vi "channel front panel validation.vi"() -> (0 "invalid_channel_class test":bool, 1 "invalid_channel_type test":bool, 2 "missing_channel_test":bool, 3 "valid channel test":bool)   [LabVIEW 2014, in "UI reference module tests.lvlib"]
uses:
  UI reference module tests.lvlib
  <vilib>/NI/Tag Bus/tag/Data Type.ctl
  <vilib>/NI/Tag Bus Module Framework/channel/channel classification.ctl
  <vilib>/NI/Tag Bus Module Framework/channel/TBM channel.lvclass
  module/execution/UI Reference runtime old.lvclass
  <vilib>/NI/Tag Bus/tag/tag descriptor.lvclass
panel:
  in  "invalid_channel_class":dbl
  in  "valid_channel_name_2":dbl
  in  "invalid_channel_type":string
  in  "valid_channel_name":dbl
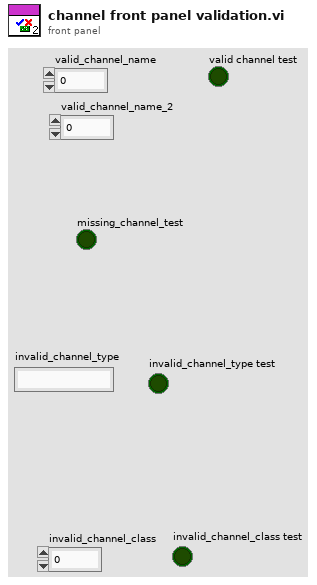
[diagram p1: front panel]
types:
  T1 = typedef "tag bus.lvlib/tag descriptor.lvclass/Data Type.ctl" = enum16{"Double", "Single", "I64", "I32", "I16", "I8", "U64", "U32", "U16", "U8", "Boolean", "String", "Array of Double", "Array of Single", "Array of I64", "Array of I32", "Array of I16", "Array of I8", "Array of U64", "Array of U32", "Array of U16", "Array of U8", "Array of Boolean", "Array of String"}
  T2 = typedef "TBM channel.lvclass/channel classification.ctl" = enum16{"input data", "output data", "processing parameter", "processing result"}
  T3 = cluster{"channel name":string, "data type":T1, "channel classification":T2}[]
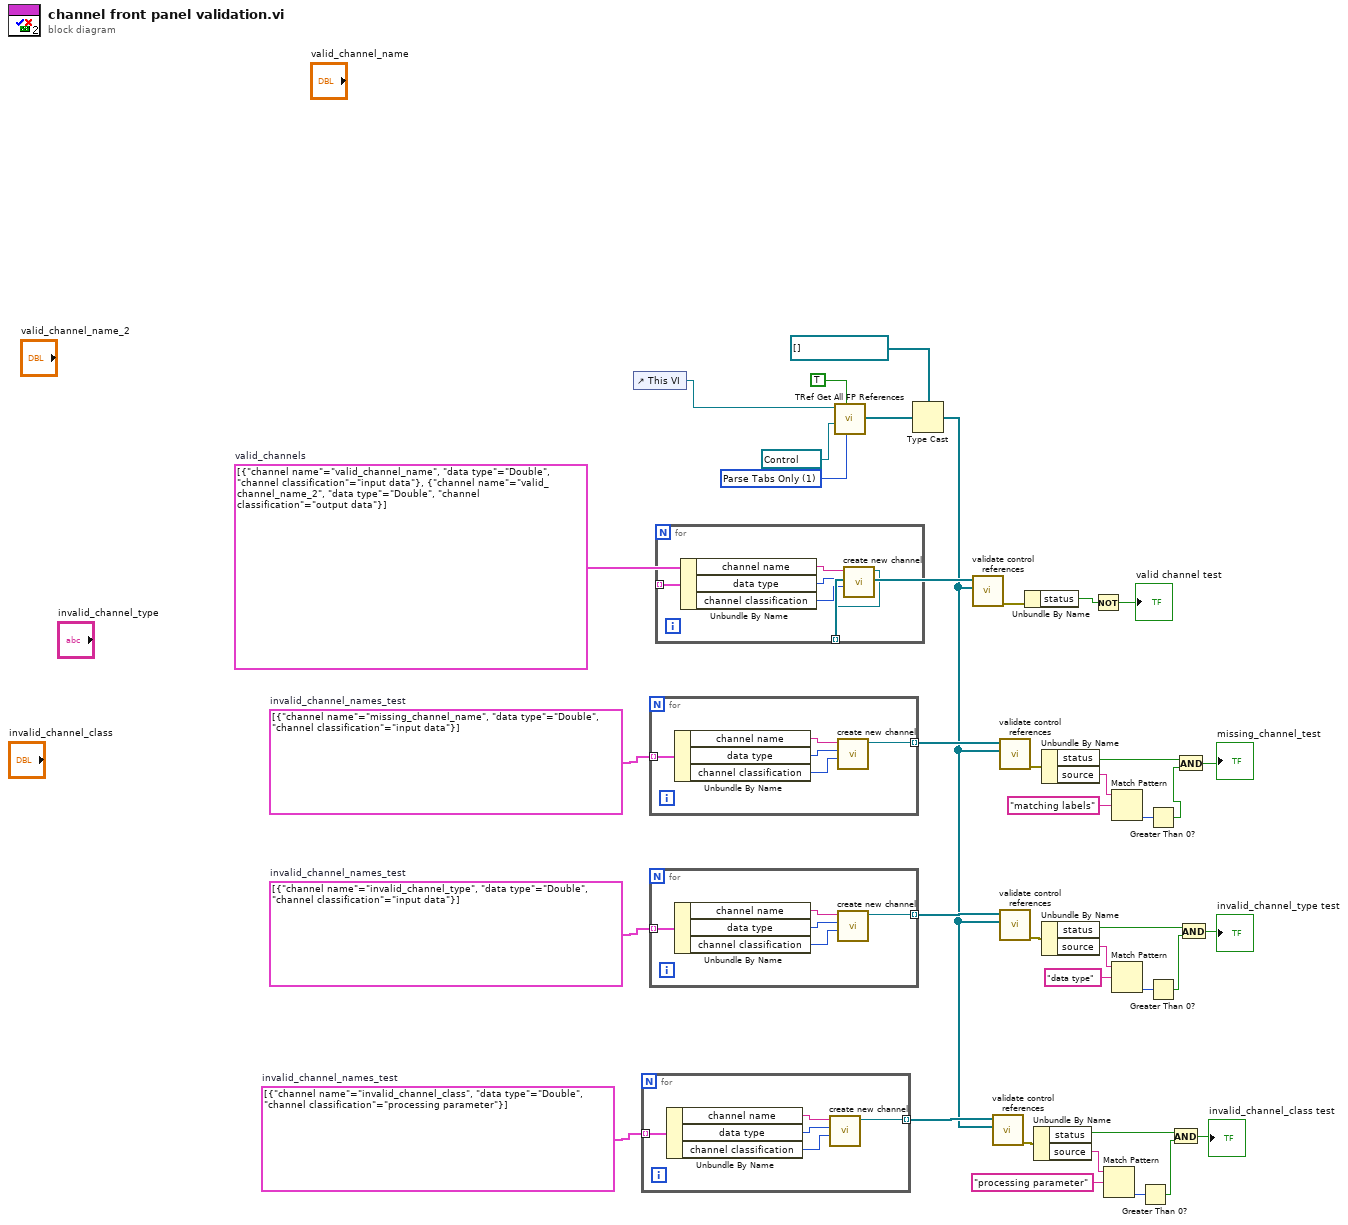
[diagram p0: block diagram]
diagram:
  w7 = T3 [{"channel name"="invalid_channel_class", "data type"=enum."Double", "channel classification"=enum."processing parameter"}]  # invalid_channel_names_test
  w17 = T3 [{"channel name"="invalid_channel_type", "data type"=enum."Double", "channel classification"=enum."input data"}]  # invalid_channel_names_test
  w28 = T3 [{"channel name"="missing_channel_name", "data type"=enum."Double", "channel classification"=enum."input data"}]  # invalid_channel_names_test
  w33 = T3 [{"channel name"="valid_channel_name", "data type"=enum."Double", "channel classification"=enum."input data"}, {"channel name"="valid_channel_name_2", "data type"=enum."Double", "channel classification"=enum."output data"}]  # valid_channels
  w38 = u16 1 items=["Parse All", "Parse Tabs Only"] ("Parsing Rule")
  n1 = control-ref of="This VI"() -> (w34:refnum<vi>)
  n2 = for {
    tunnel: w7 -> [w41] mode=indexing
    tunnel: [w40] -> w5 mode=indexing
    n3 = Unbundle By Name(w41) -> ("channel name"=w44:string, "data type"=w43:T1, "channel classification"=w42:T2)
    n4 = call <vilib>:"create new channel.vi"("channel classification"=w42, "data type"=w43, "channel name"=w44) -> ("channel"=w40:refnum<class "TBM channel.lvclass">)  [unwired: 8 in]
  }
  n5 = for {
    tunnel: w28 -> [w46] mode=indexing
    tunnel: [w45] -> w26 mode=indexing
    n6 = Unbundle By Name(w46) -> ("channel name"=w49:string, "data type"=w48:T1, "channel classification"=w47:T2)
    n7 = call <vilib>:"create new channel.vi"("channel classification"=w47, "data type"=w48, "channel name"=w49) -> ("channel"=w45:refnum<class "TBM channel.lvclass">)  [unwired: 8 in]
  }
  n8 = for {
    tunnel: w17 -> [w51] mode=indexing
    tunnel: [w50] -> w19 mode=indexing
    n9 = Unbundle By Name(w51) -> ("channel name"=w54:string, "data type"=w53:T1, "channel classification"=w52:T2)
    n10 = call <vilib>:"create new channel.vi"("channel classification"=w52, "data type"=w53, "channel name"=w54) -> ("channel"=w50:refnum<class "TBM channel.lvclass">)  [unwired: 8 in]
  }
  n11 = for {
    tunnel: w33 -> [w56] mode=indexing
    tunnel: [w55] -> w32 mode=indexing
    n12 = Unbundle By Name(w56) -> ("channel name"=w59:string, "data type"=w58:T1, "channel classification"=w57:T2)
    n13 = call <vilib>:"create new channel.vi"("channel classification"=w57, "data type"=w58, "channel name"=w59) -> ("channel"=w55:refnum<class "TBM channel.lvclass">)  [unwired: 8 in]
  }
  n14 = call <vilib>:"TRef Get All FP References.vi"("Parsing Rule"=w38, "Ignore Decorations?"=TRUE, "GObj Refnum"=refnum<vi> refnum ("Ctl Refnum"), "VI Refnum"=w34) -> ("All FP Objects"=w36:refnum<vi>[])  [unwired: 3 in, 4 out]
  n15 = Type Cast(type=refnum<vi>[] [] ("front panel elements in"), x=w36) -> (*(type *) &x=w1:refnum<vi>[])
  n16 = call "validate control references.vi"("front panel elements in"=w1, "channels in"=w32) -> ("error out"=w31:errorcluster)  [unwired: 9 in]
  n17 = call "validate control references.vi"("front panel elements in"=w1, "channels in"=w5) -> ("error out"=w6:errorcluster)  [unwired: 9 in]
  n18 = call "validate control references.vi"("front panel elements in"=w1, "channels in"=w26) -> ("error out"=w27:errorcluster)  [unwired: 9 in]
  n19 = call "validate control references.vi"("front panel elements in"=w1, "channels in"=w19) -> ("error out"=w18:errorcluster)  [unwired: 9 in]
  n20 = Unbundle By Name(w31) -> ("status"=w30:bool)
  n21 = Unbundle By Name(w6) -> ("status"=w9:bool, "source"=w4:string)
  n22 = Unbundle By Name(w27) -> ("status"=w16:bool, "source"=w25:string)
  n23 = Unbundle By Name(w18) -> ("status"=w12:bool, "source"=w20:string)
  n24 = Not(x=w30) -> (.not. x?=→"valid channel test":bool)
  n25 = Match Pattern(string=w4, regular expression="processing parameter") -> (offset past match=w2:i32)  [unwired: 1 in, 3 out]
  n26 = Match Pattern(string=w25, regular expression="matching labels") -> (offset past match=w23:i32)  [unwired: 1 in, 3 out]
  n27 = Match Pattern(string=w20, regular expression="data type") -> (offset past match=w22:i32)  [unwired: 1 in, 3 out]
  n28 = Greater Than 0?(x=w2) -> (x > 0?=w10:bool)
  n29 = Greater Than 0?(x=w23) -> (x > 0?=w15:bool)
  n30 = Greater Than 0?(x=w22) -> (x > 0?=w11:bool)
  n31 = And(x=w9, y=w10) -> (x .and. y?=→"invalid_channel_class test":bool)
  n32 = And(x=w16, y=w15) -> (x .and. y?=→"missing_channel_test":bool)
  n33 = And(x=w12, y=w11) -> (x .and. y?=→"invalid_channel_type test":bool)
